vi "Source Get Info.vi"(8 "error in":errorcluster, 11 "src in":T7={"type"=enum."Tektronix AFG3101C", "idn"="", "afg"={"VISA"="", "const"=0.0, "gen DC"=FALSE, "ext ref"=FALSE}, "cDAQ dds"={"device"="", "channels"=[], "mclk source"="", "mclk [Hz]"=0.0, "fs [Hz]"=0.0, "block [s]"=0.0, "buf [s]"=0.0, "task"="", "cmd queue"=refnum, "proc ref"=refnum, "smpl clock out"="/cDAQ3/PFI0", "export smpl clock"=FALSE, "DC ofs [V]"=[], "timebase source"="", "timebase mode"=enum."Local", "dither"=enum."Disabled", "dither level"=0.0, "phase [rad]"=[]}, "gain [V/A]"=1.0, "F5xxx session"={"VISA"="", "mode"=enum."AC voltage", "Earth on"=FALSE, "Ext ref lock"=FALSE}, "t3awg"={"VISA"="", "use ext ref"=FALSE, "ext ref [Hz]"=0.0, "load Z"=enum."High Z", "ramdac max n"=0, "noise dither [V]"=0.0, "t3awg fs rules"=[], "channels"=0, "ramdac min n"=0, "channel list"=[], "gen resl [Vpp]"=0.0, "wave data format"=enum."Binary"}} {"t3awg"."t3awg fs rules"."fs-step [Hz]" format="%#_6p"; "t3awg"."t3awg fs rules"."fs-max [Hz]" format="%#_6p"; "t3awg"."t3awg fs rules"."for f0 <" format="%#_6p"; "t3awg"."t3awg fs rules"."fs-min [Hz]" format="%#_6p"; "cDAQ dds"."channels" min=0 step=1}) -> (0 "error out":errorcluster, 2 "config info":T2, 3 "src out":T7={"type"=enum."Tektronix AFG3101C", "idn"="", "afg"={"VISA"="", "const"=0.0, "gen DC"=FALSE, "ext ref"=FALSE}, "cDAQ dds"={"device"="", "channels"=[], "mclk source"="", "mclk [Hz]"=0.0, "fs [Hz]"=0.0, "block [s]"=0.0, "buf [s]"=0.0, "task"="", "cmd queue"=refnum, "proc ref"=refnum, "smpl clock out"="/cDAQ3/PFI0", "export smpl clock"=FALSE, "DC ofs [V]"=[], "timebase source"="", "timebase mode"=enum."Local", "dither"=enum."Disabled", "dither level"=0.0, "phase [rad]"=[]}, "gain [V/A]"=1.0, "F5xxx session"={"VISA"="", "mode"=enum."AC voltage", "Earth on"=FALSE, "Ext ref lock"=FALSE}, "t3awg"={"VISA"="", "use ext ref"=FALSE, "ext ref [Hz]"=0.0, "load Z"=enum."High Z", "ramdac max n"=0, "noise dither [V]"=0.0, "t3awg fs rules"=[], "channels"=0, "ramdac min n"=0, "channel list"=[], "gen resl [Vpp]"=0.0, "wave data format"=enum."Binary"}} {"t3awg"."t3awg fs rules"."fs-step [Hz]" format="%#_6p"; "t3awg"."t3awg fs rules"."fs-max [Hz]" format="%#_6p"; "t3awg"."t3awg fs rules"."for f0 <" format="%#_6p"; "t3awg"."t3awg fs rules"."fs-min [Hz]" format="%#_6p"; "cDAQ dds"."channels" min=0 step=1})   [LabVIEW 2020]
doc: "Get text info of instrument dependent configuration."
uses:
  Source Session.ctl
  Source Type.ctl
  drivers/AFG3101C/AFG3101C Session.ctl
  drivers/cDAQ DDS/cDAQ DDS Session.ctl
  drivers/cDAQ DDS/cDAQ DDS Setup.ctl
  drivers/cDAQ DDS/cDAQ DDS Timebase Mode.ctl
  drivers/cDAQ DDS/cDAQ DDS Dither.ctl
  drivers/Fluke 5XXX/top_lev/F5xxx_session.ctl
  drivers/Fluke 5XXX/top_lev/F5xxx_output_mode.ctl
  drivers/T3AWG3K/toplevel/T3AWG Session.ctl
  drivers/T3AWG3K/toplevel/T3AWG Load Z.ctl
  drivers/T3AWG3K/toplevel/fgen_ramdac_fs_rules.ctl
  drivers/T3AWG3K/toplevel/T3AWG Channel.ctl
  Source Info.ctl
  <vilib>/ErrorRing/Error Ring.xnode
  <vilib>/Utility/error.llb/Error Cluster From Error Code.vi
  drivers/T3AWG3K/Active Technologies AWG3000.lvlib
panel:
  in  "F5xxx session.mode 2":T1
  in  "t3awg.load Z":T3
  in  "cDAQ dds.dither":T4
  in  "cDAQ dds.timebase mode":T5
  in  "F5xxx session.mode":T1
  in  "type":T6
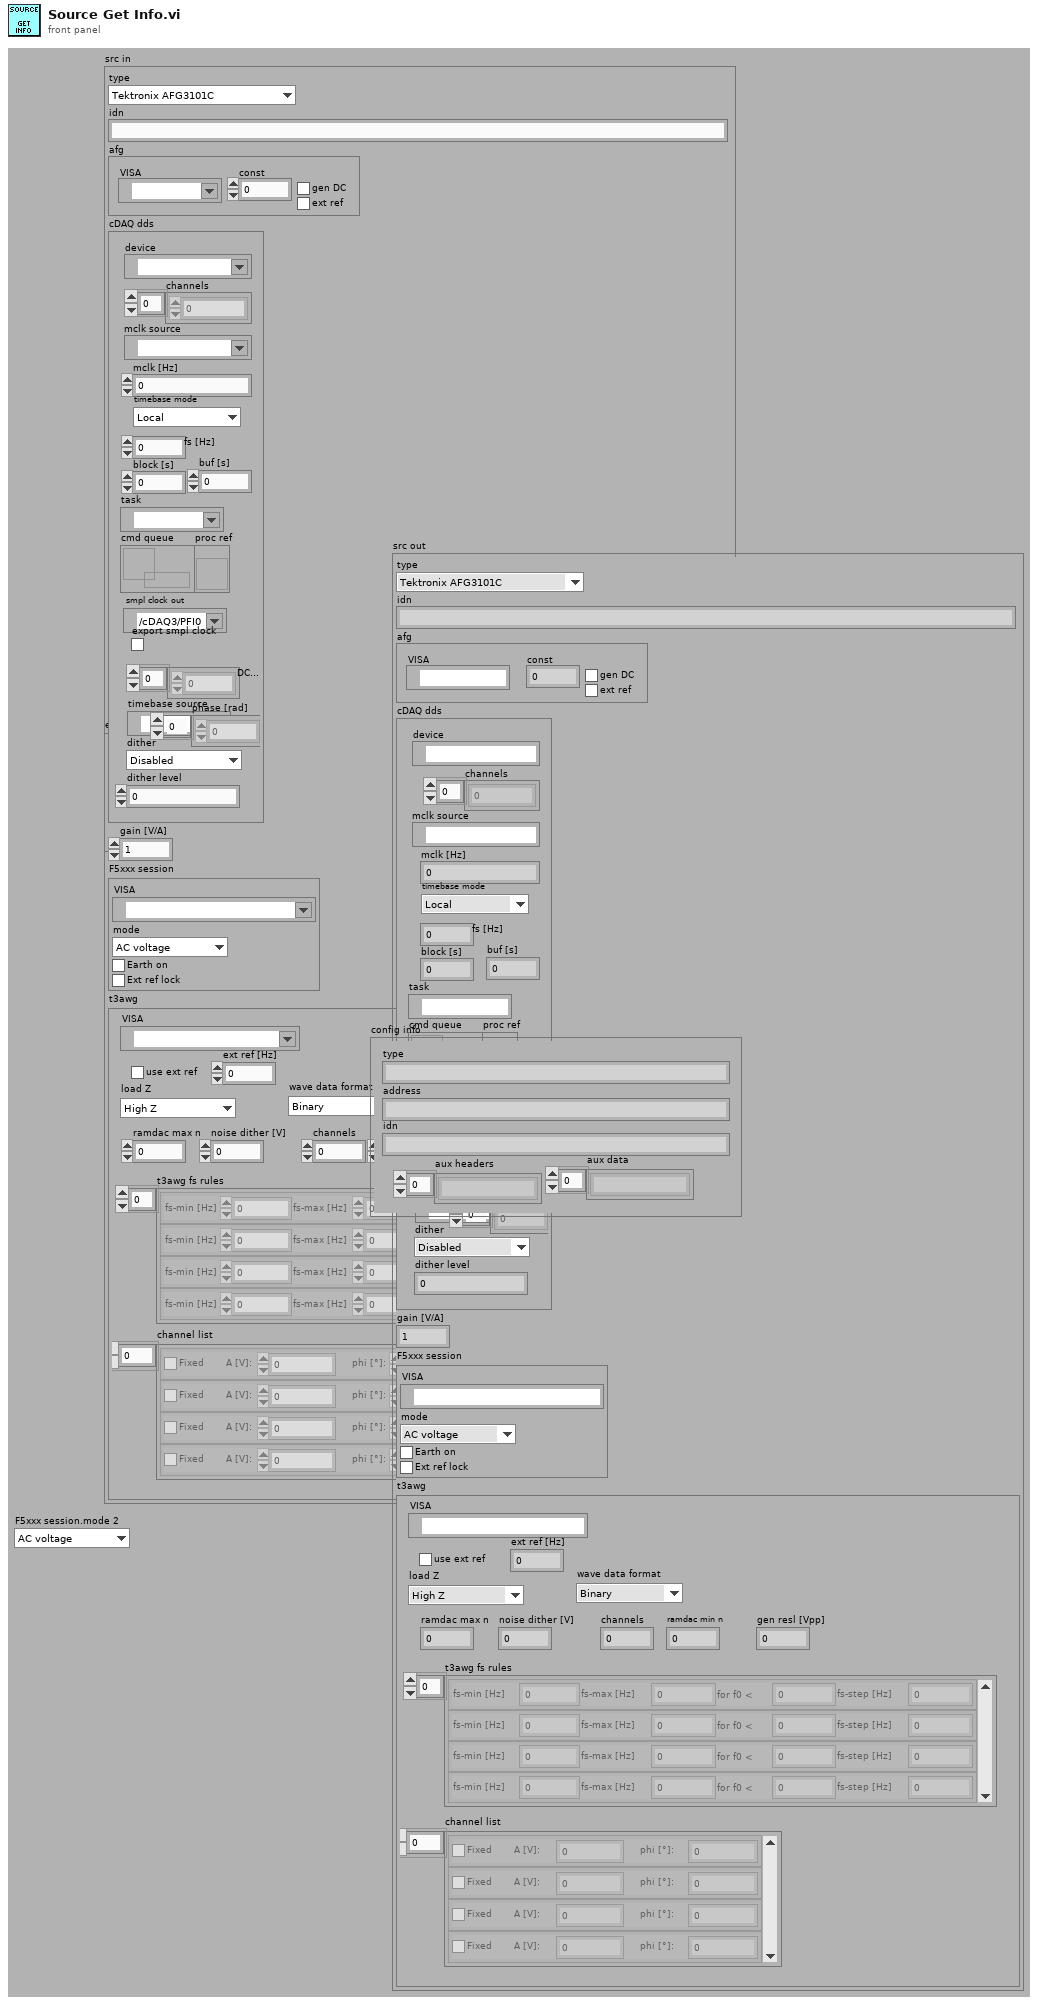
[diagram p1: front panel]
types:
  T1 = typedef "F5xxx_output_mode.ctl" = enum16{"AC voltage", "AC current"}
  T2 = typedef "Source Info.ctl" = cluster{"type":string, "address":string, "idn":string, "aux headers":string[], "aux data":string[]}
  T3 = typedef "Active Technologies AWG3000.lvlib/T3AWG Load Z.ctl" = enum16{"High Z", "50 Ohm"}
  T4 = typedef "cDAQ DDS Dither.ctl" = enum16{"Disabled", "Gaussian"}
  T5 = typedef "cDAQ DDS Timebase Mode.ctl" = enum16{"Local", "Take from ADC (e.g. NI 9238)", "Other source"}
  T6 = typedef "Source Type.ctl" = enum16{"Tektronix AFG3101C", "cDAQ DAC", "Fluke 5xxx", "Datron 4xxx", "Agilent 33120A", "R&S SMT", "Teledyne LeCroy T3AWG", "dummy"}
  T7 = typedef "Source Session.ctl" = cluster{"type":T6, "idn":string, "afg":T8, "cDAQ dds":T9, "gain [V/A]":dbl, "F5xxx session":T10, "t3awg":T11}
  T8 = typedef "AFG3101C Session.ctl" = cluster{"VISA":refnum<visa-resource-name>, "const":dbl, "gen DC":bool, "ext ref":bool}
  T9 = typedef "cDAQ DDS Session.ctl" = cluster{"device":tag, "channels":i32[], "mclk source":tag, "mclk [Hz]":dbl, "fs [Hz]":dbl, "block [s]":dbl, "buf [s]":dbl, "task":refnum<k21>, "cmd queue":refnum<queue>, "proc ref":refnum<vi>, "smpl clock out":tag, "export smpl clock":bool, "DC ofs [V]":dbl[], "timebase source":tag, "timebase mode":T5, "dither":T4, "dither level":dbl, "phase [rad]":dbl[]}
  T10 = typedef "F5xxx_session.ctl" = cluster{"VISA":refnum<visa-resource-name>, "mode":T1, "Earth on":bool, "Ext ref lock":bool}
  T11 = typedef "Active Technologies AWG3000.lvlib/T3AWG Session.ctl" = cluster{"VISA":refnum<visa-resource-name>, "use ext ref":bool, "ext ref [Hz]":dbl, "load Z":T3, "ramdac max n":i32, "noise dither [V]":dbl, "t3awg fs rules":T12[], "channels":i32, "ramdac min n":i32, "channel list":T13[], "gen resl [Vpp]":dbl, "wave data format":T14}
  T12 = typedef "Active Technologies AWG3000.lvlib/fgen_ramdac_fs_rules.ctl" = cluster{"fs-min [Hz]":dbl, "fs-max [Hz]":dbl, "for f0 < ":dbl, "fs-step [Hz]":dbl}
  T13 = typedef "Active Technologies AWG3000.lvlib/T3AWG Channel.ctl" = cluster{"Fixed":bool, "A [V]:":dbl, "phi [°]:":dbl}
  T14 = typedef "Active Technologies AWG3000.lvlib/T3AWG Wave Format" = enum16{"Text", "Binary"}
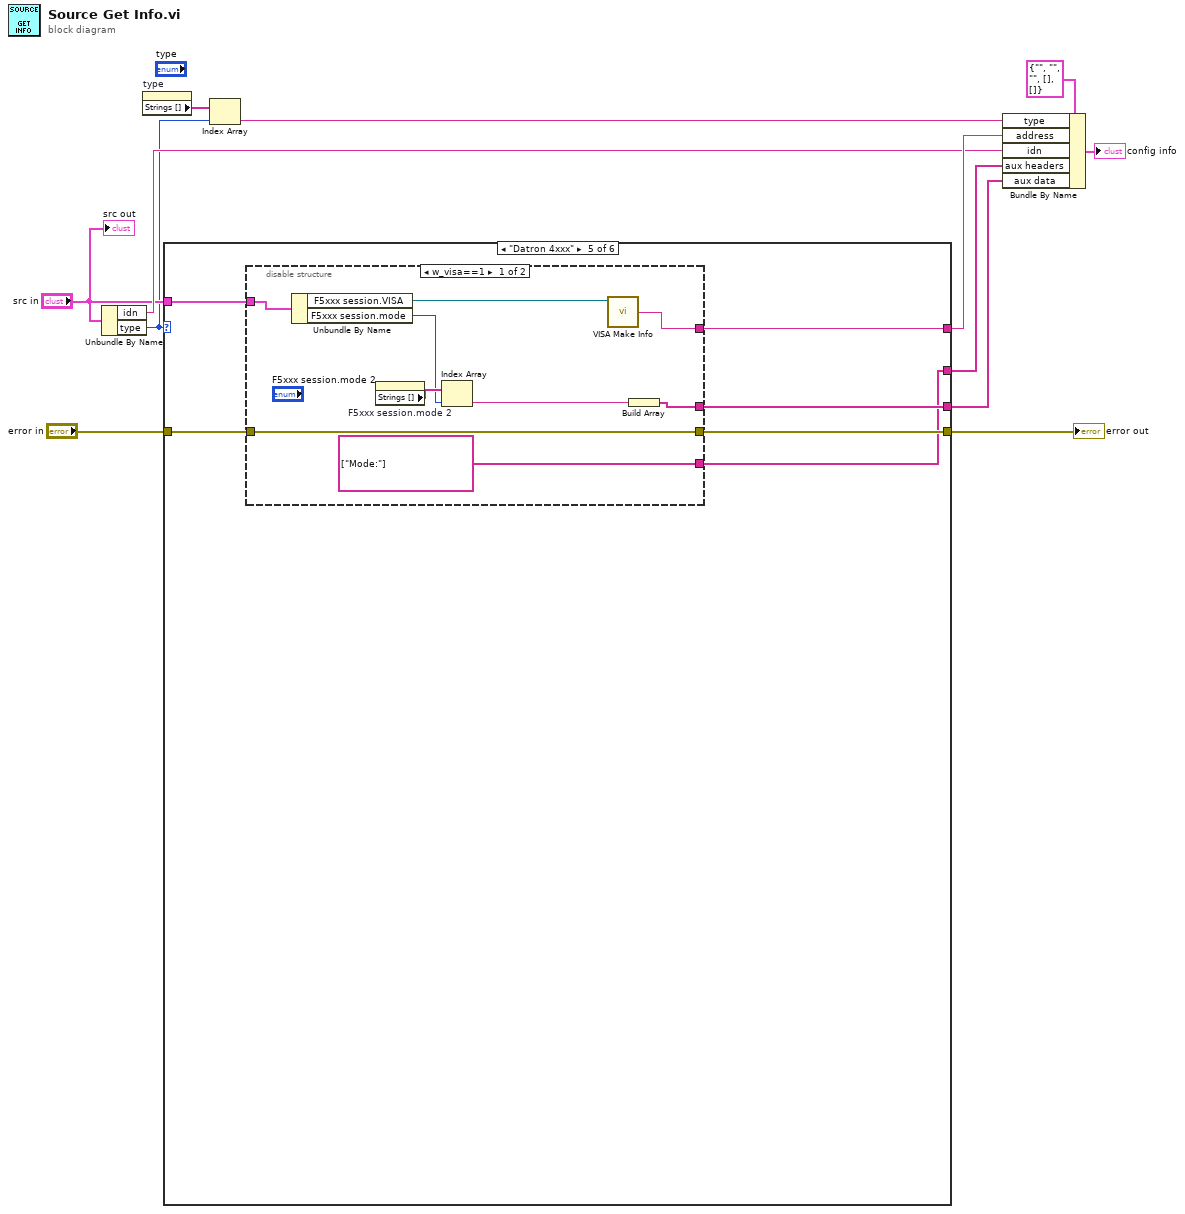
[diagram p0: block diagram]
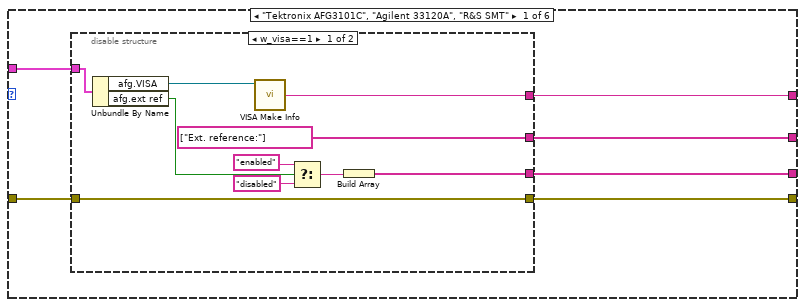
[diagram p2: hidden frame]
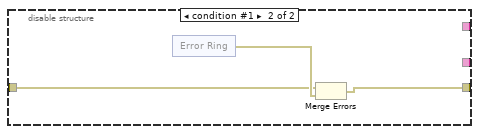
[diagram p3: hidden frame]
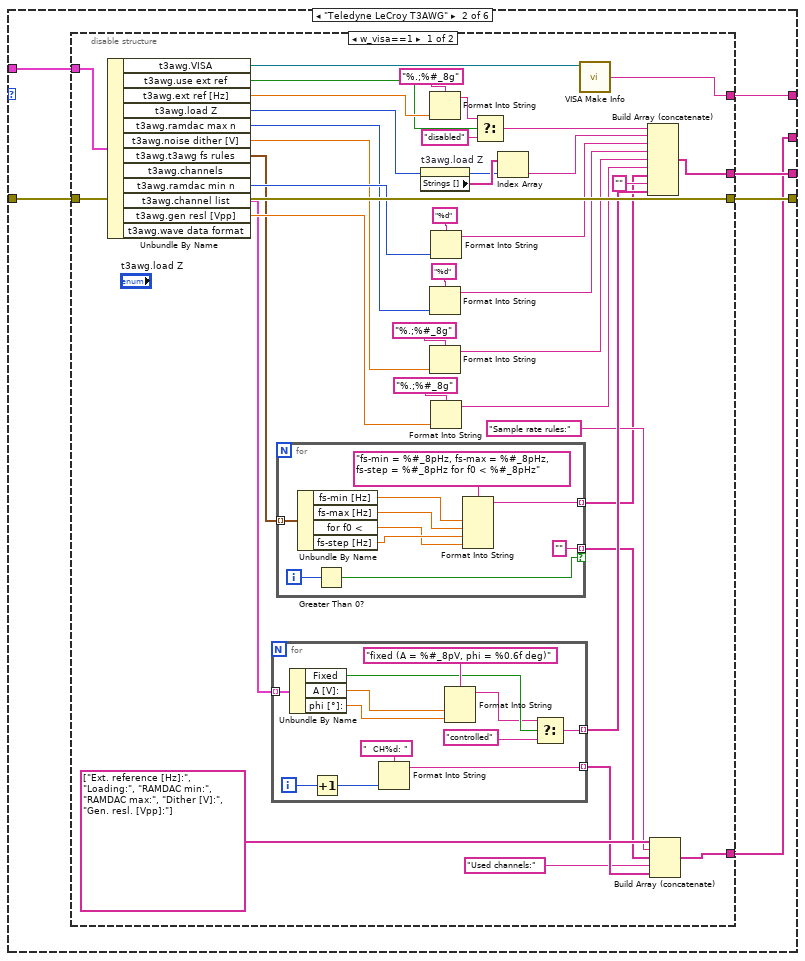
[diagram p4: hidden frame]
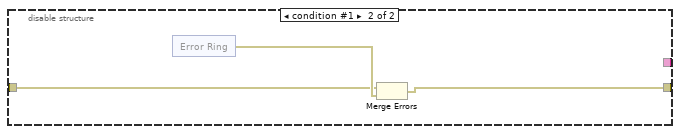
[diagram p5: hidden frame]
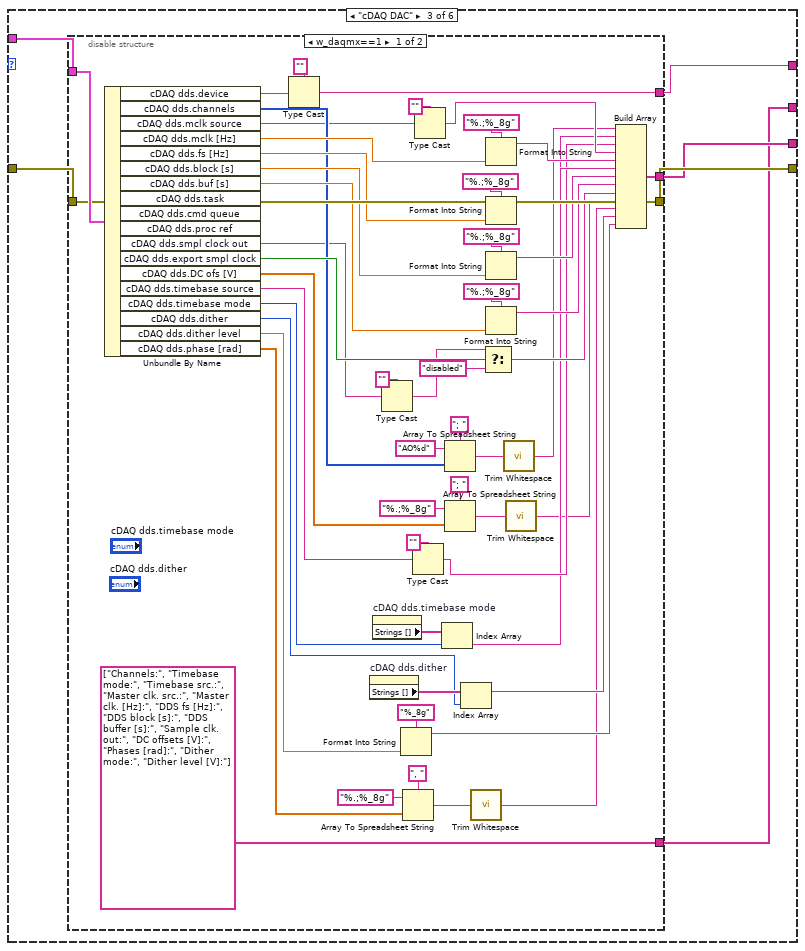
[diagram p6: hidden frame]
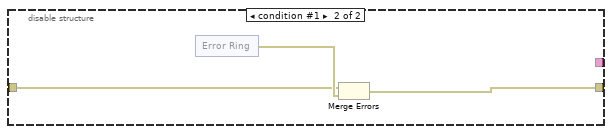
[diagram p7: hidden frame]
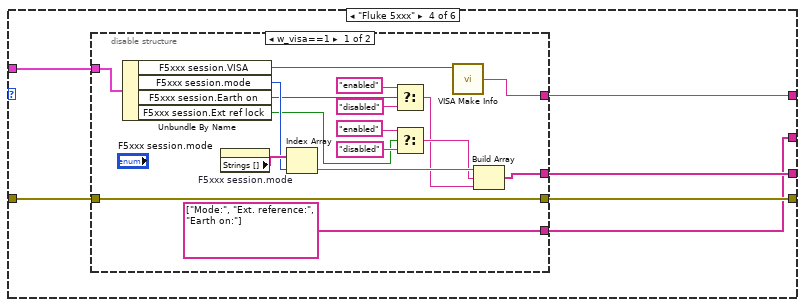
[diagram p8: hidden frame]
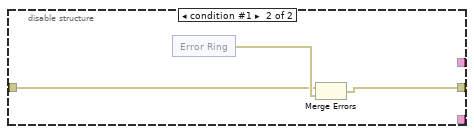
[diagram p9: hidden frame]
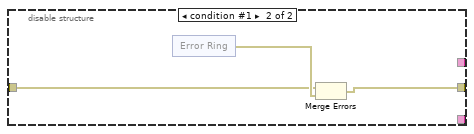
[diagram p10: hidden frame]
diagram:
  n1 = Unbundle By Name("src in") -> ("idn"=w6:string, "type"=w2:T6)
  n2 = property on="type" class="Enum (strict)"() -> ("Strings []"=w9:string[])  [unwired: 2 in, 2 out]
  n3 = case shown="\"Datron 4xxx\"" w2 {
    tunnel: "src in" -> [w18 w42 w114 w183 w214 _]
    tunnel: "error in" -> [w16 w40 w115 w184 w215 w233]
    tunnel: [w17 w41 w113 w182 w213 w233] -> w11
    tunnel: [w15 w39 w110 w181 w212 _] -> w7
    tunnel: [w14 w37 w111 w179 w210 _] -> w4
    tunnel: [w13 w38 w112 w180 w211 _] -> w3
    frame "Tektronix AFG3101C", "Agilent 33120A", "R&S SMT" {
      n4 = disable-structure shown="w_visa==1" {
        disable-tunnel: w16 -> [w24 w30]
        disable-tunnel: w18 -> [w28 _]
        disable-tunnel: [w24 w29] -> w17
        disable-tunnel: [w26 _] -> w15
        disable-tunnel: [string[] ["Ext. reference:"] ("aux headers") _] -> w14
        disable-tunnel: [w19 _] -> w13
        frame condition #0 (active) {
          n5 = Unbundle By Name(w28) -> ("afg.VISA"=w27:refnum<visa-resource-name>, "afg.ext ref"=w23:bool)
          n6 = call "VISA Make Info.vi"("VISA in"=w27) -> ("info string"=w26:string)  [unwired: 3 in]
          n7 = Select(t="enabled" ("String"), s=w23, f="disabled" ("String")) -> (s? t:f=w20:string)
          n8 = Build Array(w20) -> (w19:string[])
        }
        frame condition #1 {
          n9 = xnode "Error Ring"() -> ("error out"=w31:errorcluster)
          n10 = Merge Errors(w30, w31) -> (w29:errorcluster)
        }
      }
    }
    frame "Teledyne LeCroy T3AWG" {
      n11 = disable-structure shown="w_visa==1" {
        disable-tunnel: w40 -> [w78 w103]
        disable-tunnel: w42 -> [w79 _]
        disable-tunnel: [w78 w102] -> w41
        disable-tunnel: [w76 _] -> w39
        disable-tunnel: [w49 _] -> w38
        disable-tunnel: [w48 _] -> w37
        frame condition #0 (active) {
          n12 = Unbundle By Name(w79) -> ("t3awg.VISA"=w77:refnum<visa-resource-name>, "t3awg.use ext ref"=w71:bool, "t3awg.ext ref [Hz]"=w73:dbl, "t3awg.load Z"=w45:T3, "t3awg.ramdac max n"=w67:i32, "t3awg.noise dither [V]"=w65:dbl, "t3awg.t3awg fs rules"=w54:T12[], "t3awg.ramdac min n"=w68:i32, "t3awg.channel list"=w62:T13[], "t3awg.gen resl [Vpp]"=w63:dbl)  [unwired: 2 out]
          n13 = for {
            tunnel: w62 -> [w101] mode=indexing
            tunnel: [w92] -> w56 mode=indexing
            tunnel: [w90] -> w44 mode=indexing
            i -> [w99]
            n14 = Unbundle By Name(w101) -> ("Fixed"=w94:bool, "A [V]:"=w96:dbl, "phi [°]:"=w95:dbl)
            n15 = Increment(x=w99) -> (x+1=w97:i32)
            n16 = Format Into String(format string="  CH%d: ", w97) -> (resulting string=w90:string)  [unwired: 2 in, 1 out]
            n17 = Format Into String(format string="fixed (A = %#_8pV, phi = %0.6f deg)", w96, w95) -> (resulting string=w93:string)  [unwired: 2 in, 1 out]
            n18 = Select(t=w93, s=w94, f="controlled" ("string")) -> (s? t:f=w92:string)
          }
          n19 = for {
            tunnel: w54 -> [w89] mode=indexing
            tunnel: [w83] -> w50 mode=indexing
            tunnel: ["" ("format string")] -> w52 mode=indexing if=w80
            i -> [w81]
            n20 = Unbundle By Name(w89) -> ("fs-min [Hz]"=w87:dbl, "fs-max [Hz]"=w86:dbl, "for f0 <"=w84:dbl, "fs-step [Hz]"=w85:dbl)
            n21 = Greater Than 0?(x=w81) -> (x > 0?=w80:bool)
            n22 = Format Into String(format string="fs-min = %#_8pHz, fs-max = %#_8pHz, fs-step = %#_8pHz for f0 < %#_8pHz", w87, w86, w85, w84) -> (resulting string=w83:string)  [unwired: 2 in, 1 out]
          }
          n23 = property on="t3awg.load Z" class="Enum (strict)"() -> ("Strings []"=w47:string[])  [unwired: 2 in, 2 out]
          n24 = Format Into String(format string="%.;%#_8g", w73) -> (resulting string=w72:string)  [unwired: 2 in, 1 out]
          n25 = Format Into String(format string="%d", w67) -> (resulting string=w59:string)  [unwired: 2 in, 1 out]
          n26 = Format Into String(format string="%.;%#_8g", w65) -> (resulting string=w58:string)  [unwired: 2 in, 1 out]
          n27 = Format Into String(format string="%d", w68) -> (resulting string=w60:string)  [unwired: 2 in, 1 out]
          n28 = Format Into String(format string="%.;%#_8g", w63) -> (resulting string=w57:string)  [unwired: 2 in, 1 out]
          n29 = Select(t=w72, s=w71, f="disabled") -> (s? t:f=w61:string)
          n30 = Index Array(array=w47, index=w45) -> (element=w46:string)
          n31 = call "VISA Make Info.vi"("VISA in"=w77) -> ("info string"=w76:string)  [unwired: 3 in]
          n32 = Build Array (concatenate)(w61, w46, w60, w59, w58, w57, w50, "" ("element"), w56) -> (w49:string[])
          n33 = Build Array (concatenate)(string[] ["Ext. reference [Hz]:", "Loading:", "RAMDAC min:", "RAMDAC max:", "Dither [V]:", "Gen. resl. [Vpp]:"] ("aux headers"), "Sample rate rules:" ("String"), w52, "Used channels:" ("String"), w44) -> (w48:string[])
        }
        frame condition #1 {
          n34 = xnode "Error Ring"() -> ("error out"=w104:errorcluster)
          n35 = Merge Errors(w103, w104) -> (w102:errorcluster)
        }
      }
    }
    frame "cDAQ DAC" {
      n36 = disable-structure shown="w_daqmx==1" {
        disable-tunnel: w115 -> [w169 w172]
        disable-tunnel: w114 -> [w170 _]
        disable-tunnel: [w169 w171] -> w113
        disable-tunnel: [w166 _] -> w110
        disable-tunnel: [w133 _] -> w112
        disable-tunnel: [string[] ["Channels:", "Timebase mode:", "Timebase src.:", "Master clk. src.:", "Master clk. [Hz]:", "DDS fs [Hz]:", "DDS block [s]:", "DDS buffer [s]:", "Sample clk. out:", "DC offsets [V]:", "Phases [rad]:", "Dither mode:", "Dither level [V]:"] ("aux headers") _] -> w111
        frame condition #0 (active) {
          n37 = Unbundle By Name(w170) -> ("cDAQ dds.device"=w168:tag, "cDAQ dds.channels"=w155:i32[], "cDAQ dds.mclk source"=w130:tag, "cDAQ dds.mclk [Hz]"=w165:dbl, "cDAQ dds.fs [Hz]"=w162:dbl, "cDAQ dds.block [s]"=w160:dbl, "cDAQ dds.buf [s]"=w158:dbl, "cDAQ dds.smpl clock out"=w127:tag, "cDAQ dds.export smpl clock"=w157:bool, "cDAQ dds.DC ofs [V]"=w150:dbl[], "cDAQ dds.timebase source"=w124:tag, "cDAQ dds.timebase mode"=w121:T5, "cDAQ dds.dither"=w119:T4, "cDAQ dds.dither level"=w148:dbl, "cDAQ dds.phase [rad]"=w146:dbl[])  [unwired: 3 out]
          n38 = Type Cast(type="", x=w168) -> (*(type *) &x=w166:string)
          n39 = property on="cDAQ dds.dither" class="Enum (strict)"() -> ("Strings []"=w135:string[])  [unwired: 2 in, 2 out]
          n40 = property on="cDAQ dds.timebase mode" class="Enum (strict)"() -> ("Strings []"=w143:string[])  [unwired: 2 in, 2 out]
          n41 = Type Cast(type="", x=w127) -> (*(type *) &x=w126:string)
          n42 = Format Into String(format string="%_8g", w148) -> (resulting string=w134:string)  [unwired: 2 in, 1 out]
          n43 = Array To Spreadsheet String(delimiter (Tab)=", ", array=w146, 3:"%.;%_8g" ("format string")) -> (spreadsheet string=w136:string)
          n44 = Type Cast(type="", x=w124) -> (*(type *) &x=w123:string)
          n45 = Type Cast(type="", x=w130) -> (*(type *) &x=w129:string)
          n46 = Index Array(array=w143, index=w121) -> (element=w122:string)
          n47 = Array To Spreadsheet String(delimiter (Tab)="; ", array=w155, 3:"AO%d" ("format string")) -> (spreadsheet string=w144:string)
          n48 = Array To Spreadsheet String(delimiter (Tab)="; ", array=w150, 3:"%.;%_8g" ("format string")) -> (spreadsheet string=w137:string)
          n49 = Index Array(array=w135, index=w119) -> (element=w120:string)
          n50 = call <vilib>:"Trim Whitespace.vi"("string"=w136) -> ("trimmed string"=w116:string)  [unwired: 1 in]
          n51 = Select(t=w126, s=w157, f="disabled") -> (s? t:f=w138:string)
          n52 = Format Into String(format string="%.;%_8g", w165) -> (resulting string=w142:string)  [unwired: 2 in, 1 out]
          n53 = Format Into String(format string="%.;%_8g", w162) -> (resulting string=w141:string)  [unwired: 2 in, 1 out]
          n54 = Format Into String(format string="%.;%_8g", w160) -> (resulting string=w140:string)  [unwired: 2 in, 1 out]
          n55 = Format Into String(format string="%.;%_8g", w158) -> (resulting string=w139:string)  [unwired: 2 in, 1 out]
          n56 = call <vilib>:"Trim Whitespace.vi"("string"=w144) -> ("trimmed string"=w118:string)  [unwired: 1 in]
          n57 = call <vilib>:"Trim Whitespace.vi"("string"=w137) -> ("trimmed string"=w117:string)  [unwired: 1 in]
          n58 = Build Array(w118, w122, w123, w129, w142, w141, w140, w139, w138, w117, w116, w120, w134) -> (w133:string[])
        }
        frame condition #1 {
          n59 = xnode "Error Ring"() -> ("error out"=w173:errorcluster)
          n60 = Merge Errors(w172, w173) -> (w171:errorcluster)
        }
      }
    }
    frame "Fluke 5xxx" {
      n61 = disable-structure shown="w_visa==1" {
        disable-tunnel: w184 -> [w196 w203]
        disable-tunnel: w183 -> [w201 _]
        disable-tunnel: [w196 w202] -> w182
        disable-tunnel: [w199 _] -> w181
        disable-tunnel: [w186 _] -> w180
        disable-tunnel: [string[] ["Mode:", "Ext. reference:", "Earth on:"] ("aux headers") _] -> w179
        frame condition #0 (active) {
          n62 = Unbundle By Name(w201) -> ("F5xxx session.VISA"=w200:refnum<visa-resource-name>, "F5xxx session.mode"=w197:T1, "F5xxx session.Earth on"=w192:bool, "F5xxx session.Ext ref lock"=w189:bool)
          n63 = property on="F5xxx session.mode" class="Enum (strict)"() -> ("Strings []"=w198:string[])  [unwired: 2 in, 2 out]
          n64 = Index Array(array=w198, index=w197) -> (element=w195:string)
          n65 = Select(t="enabled" ("String"), s=w192, f="disabled" ("String")) -> (s? t:f=w187:string)
          n66 = Select(t="enabled" ("String"), s=w189, f="disabled" ("String")) -> (s? t:f=w188:string)
          n67 = call "VISA Make Info.vi"("VISA in"=w200) -> ("info string"=w199:string)  [unwired: 3 in]
          n68 = Build Array(w195, w188, w187) -> (w186:string[])
        }
        frame condition #1 {
          n69 = xnode "Error Ring"() -> ("error out"=w204:errorcluster)
          n70 = Merge Errors(w203, w204) -> (w202:errorcluster)
        }
      }
    }
    frame "Datron 4xxx" {
      n71 = disable-structure shown="w_visa==1" {
        disable-tunnel: w215 -> [w219 w226]
        disable-tunnel: w214 -> [w224 _]
        disable-tunnel: [w219 w225] -> w213
        disable-tunnel: [w222 _] -> w212
        disable-tunnel: [w217 _] -> w211
        disable-tunnel: [string[] ["Mode:"] ("aux headers") _] -> w210
        frame condition #0 (active) {
          n72 = Unbundle By Name(w224) -> ("F5xxx session.VISA"=w223:refnum<visa-resource-name>, "F5xxx session.mode"=w220:T1)
          n73 = property on="F5xxx session.mode 2" class="Enum (strict)"() -> ("Strings []"=w221:string[])  [unwired: 2 in, 2 out]
          n74 = Index Array(array=w221, index=w220) -> (element=w218:string)
          n75 = call "VISA Make Info.vi"("VISA in"=w223) -> ("info string"=w222:string)  [unwired: 3 in]
          n76 = Build Array(w218) -> (w217:string[])
        }
        frame condition #1 {
          n77 = xnode "Error Ring"() -> ("error out"=w227:errorcluster)
          n78 = Merge Errors(w226, w227) -> (w225:errorcluster)
        }
      }
    }
    frame "dummy", Default {
    }
  }
  "error out" <- w11
  n79 = Index Array(array=w9, index=w2) -> (element=w8:string)
  n80 = Bundle By Name(cluster=T2 {"type"="", "address"="", "idn"="", "aux headers"=[], "aux data"=[]} ("source info"), "type"=w8, "address"=w7, "idn"=w6, "aux headers"=w4, "aux data"=w3) -> (→"config info":T2)
  "src out" <- "src in"
